vi "I_Sense_v3b.vi"(8 "error in":errorcluster, 9 "Test Freq":enum16{"10Hz", "1kHz", "20kHz"}(ring), 10 "Write Channel(s)":string="NI9264/ao2") -> (0 "error out":errorcluster, 3 "Result":dbl[](array[numeric]))   [LabVIEW 2021]
uses:
  <vilib>/DAQmx/write.llb/DAQmx Write (Analog 1D Wfm NChan NSamp).vi
  <vilib>/DAQmx/read.llb/DAQmx Read (Analog 1D Wfm NChan NSamp).vi
  <vilib>/DAQmx/create/channels.llb/DAQmx Create Channel (AO-Voltage-Basic).vi
  <vilib>/DAQmx/create/channels.llb/DAQmx Create Channel (AI-Voltage-Basic).vi
  <vilib>/DAQmx/configure/timing.llb/DAQmx Timing (Sample Clock).vi
  <vilib>/measure/mascope.llb/Amplitude and Levels N chan.vi
  <vilib>/DAQmx/miscellaneous.llb/DAQmx Fill In Error Info.vi
  <vilib>/measure/madcrms.llb/Basic Averaged DC-RMS for N Chan.vi
  <resource>/objmgr/daqmx.rc
  <vilib>/measure/NI_MABase.lvlib
  <vilib>/measure/NI_MAPro.lvlib
panel:
  in  "Cycles":i32=4
  in  "Read Channel(s)":string="BONTS_ISENSE"
  out "DC values":dbl[](array[numeric]) format="%.2p"
  out "Gains":dbl[](array[numeric])
  out "Amplitude Out":dbl[](array[numeric]) format="%.2p"
  out "High Out":dbl[](array[numeric]) format="%.2p"
  out "Low Out":dbl[](array[numeric]) format="%.2p"
  out "Amplitude In":dbl[](array[numeric]) format="%.2p"
  out "Low In":dbl[](array[numeric]) format="%.2p"
  out "High In":dbl[](array[numeric]) format="%.2p"
  in  "Sample Mode":i32(ring)=10123 items=["Finite Samples"=10178, "Continuous Samples"=10123, "Hardware Timed Single Point"=12522]
  out "Output Waveform":waveform(dbl)[](graph)=[{"t0"=timestamp(0 s since 1904-01-01), "dt"=0.001, "Y"=[]}]
  out "Input Waveform":waveform(dbl)[](graph)=[{"t0"=timestamp(0 s since 1904-01-01), "dt"=0.001, "Y"=[]}]
  in  "Sample Clock Source":tag="OnboardClock"
  out "Actual Sample Rate":dbl=1000.0 format="%0.2f"
  # "ISENSE_C+"
  # "ISENSE_C-"
  # "ISENSE_C+"
  # "ISENSE_C-"
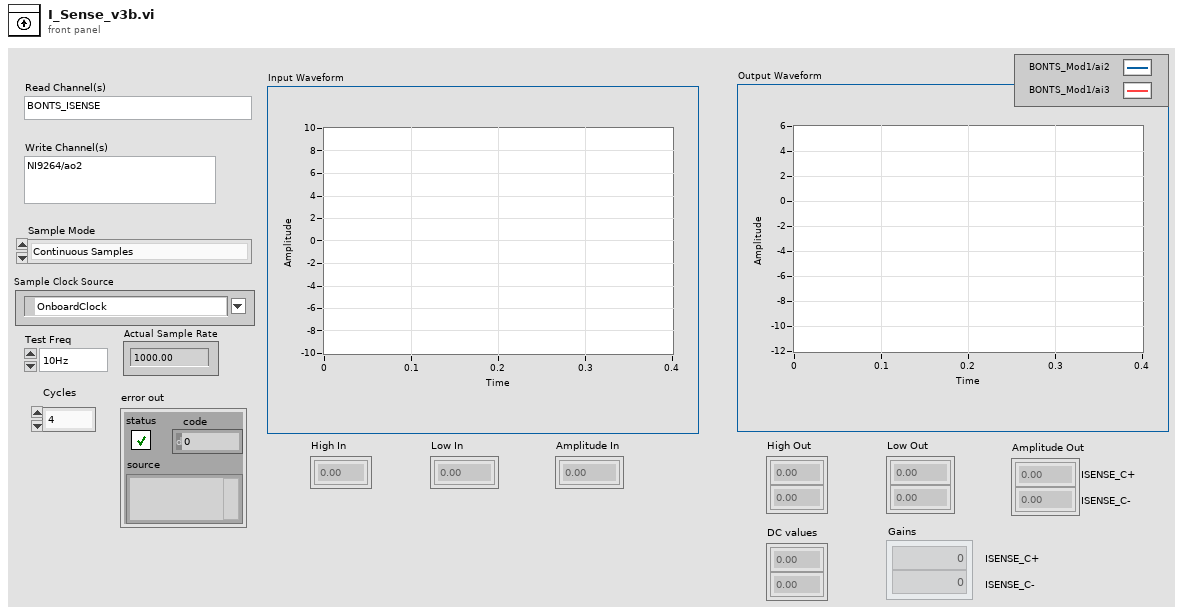
[diagram p1: front panel]
types:
  T1 = cluster{"Waveform Type":u16, "Amplitude":dbl, "Frequency":dbl}[]
  T2 = cluster{"Waveform Type":u16, "Amplitude":dbl, "Frequency":dbl}
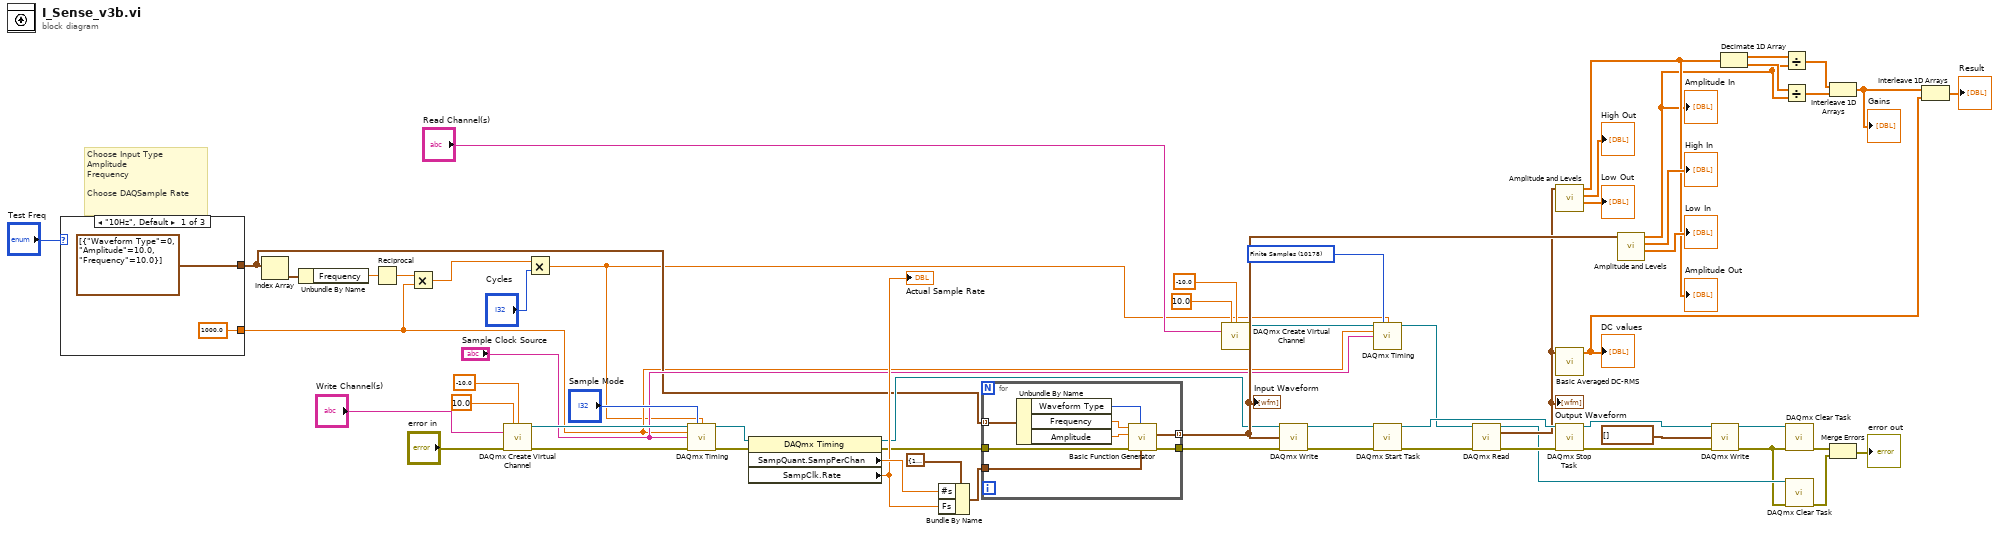
[diagram p0: block diagram]
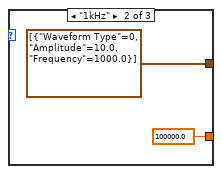
[diagram p2: hidden frame]
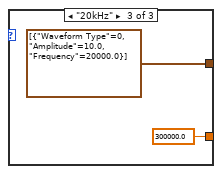
[diagram p3: hidden frame]
diagram:
  w16 = 10178 items=["Finite Samples"=10178, "Continuous Samples"=10123, "Hardware Timed Single Point"=12522] ("sample mode")
  # "Choose Input Type\nAmplitude \nFrequency\n\nChoose DAQSample Rate"
  n1 = case shown="\"10Hz\", Default" "Test Freq" {
    tunnel: [1000.0 ("Sample Rate") 100000.0 ("Sample Rate") 300000.0 ("Sample Rate")] -> w4
    tunnel: [T1 [{"Waveform Type"=0, "Amplitude"=10.0, "Frequency"=10.0}] ("Output Array") T1 [{"Waveform Type"=0, "Amplitude"=10.0, "Frequency"=1000.0}] ("Output Array") T1 [{"Waveform Type"=0, "Amplitude"=10.0, "Frequency"=20000.0}] ("Output Array")] -> w8
    frame "10Hz", Default {
    }
    frame "1kHz" {
    }
    frame "20kHz" {
    }
  }
  n2 = Index Array(array=w8) -> (element=w7:T2)  [unwired: 1 in]
  n3 = Unbundle By Name(w7) -> ("Frequency"=w6:dbl)
  n4 = Reciprocal(x=w6) -> (1/x=w5:dbl)
  n5 = Multiply(x=w5, y=w4) -> (x*y=w3:dbl)
  n6 = call-poly <vilib>:"DAQmx Create Virtual Channel.vi"("maximum value"=10.0, "minimum value"=-10.0, "physical channels"="Write Channel(s)", "error in"="error in") -> ("task out"=w58:refnum<k21>, "error out"=w59:errorcluster)  [unwired: 10 in]
  n7 = Multiply(x=w3, y="Cycles") -> (x*y=w2:dbl)
  n8 = call-poly <vilib>:"DAQmx Timing.vi"("task/channels in"=w58, "sample mode"="Sample Mode", "samples per channel"=w2, "rate"=w4, "source"="Sample Clock Source", "error in"=w59) -> ("task out"=w28:refnum<k21>, "error out"=w61:errorcluster)  [unwired: 8 in]
  n9 = property class="DAQmx Timing"(reference=w28, error in=w61) -> (reference out=w25:refnum<k21>, error out=w49:errorcluster, "SampQuant.SampPerChan"=w52:dbl, "SampClk.Rate"=w51:dbl)
  "Actual Sample Rate" <- w51
  n10 = Bundle By Name(cluster=cluster{"Fs":dbl, "#s":dbl} {"Fs"=1000.0, "#s"=1000.0} ("sampling info"), "#s"=w52, "Fs"=w51) -> (w56:cluster{"Fs":dbl, "#s":dbl})
  n11 = for {
    tunnel: w49 -> [w75]
    tunnel: w56 -> [w74]
    tunnel: [w73] -> w53
    tunnel: w8 -> [w72] mode=indexing
    tunnel: [w68] -> w44 mode=indexing
    n12 = Unbundle By Name(w72) -> ("Waveform Type"=w71:u16, "Frequency"=w70:dbl, "Amplitude"=w69:dbl)
    n13 = call <vilib>:"Basic Function Generator.vi"("sampling info"=w74, "signal type"=w71, "error in (no error)"=w75, "amplitude"=w69, "frequency"=w70) -> ("error out"=w73:errorcluster, "signal out"=w68:waveform(dbl))  [unwired: 4 in, 1 out]
  }
  "Input Waveform" <- w44
  n14 = call-poly <vilib>:"DAQmx Create Virtual Channel.vi"("maximum value"=10.0, "minimum value"=-10.0, "physical channels"="Read Channel(s)") -> ("task out"=w20:refnum<k21>)  [unwired: 11 in, 1 out]
  n15 = call-poly <vilib>:"DAQmx Write.vi"("task/channels in"=w25, "data"=w44, "error in"=w53) -> ("task out"=w55:refnum<k21>, "error out"=w54:errorcluster)  [unwired: 10 in, 1 out]
  n16 = call-poly <vilib>:"DAQmx Timing.vi"("task/channels in"=w20, "sample mode"=w16, "samples per channel"=w2, "rate"=w4, "source"="Sample Clock Source") -> ("task out"=w19:refnum<k21>)  [unwired: 9 in, 1 out]
  n17 = call <vilib>:"DAQmx Start Task.vi"("task/channels in"=w55, "error in"=w54) -> ("task out"=w50:refnum<k21>, "error out"=w48:errorcluster)  [unwired: 12 in]
  n18 = call-poly <vilib>:"DAQmx Read.vi"("task/channels in"=w19, "error in"=w48) -> ("task out"=w18:refnum<k21>, "data"=w32:waveform(dbl)[], "error out"=w47:errorcluster)  [unwired: 11 in]
  "Output Waveform" <- w32
  n19 = call-poly <vilib>:"Amplitude and Levels.vi"("signal(s) in"=w32) -> ("low state level"=→"Low Out":dbl[], "high state level"=→"High Out":dbl[], "amplitude"=w38:dbl[])  [unwired: 7 in, 1 out]
  "Amplitude Out" <- w38
  n20 = call-poly <vilib>:"Basic Averaged DC-RMS.vi"("signals in"=w32) -> ("DC values"=w30:dbl[])  [unwired: 7 in, 3 out]
  "DC values" <- w30
  n21 = call <vilib>:"DAQmx Stop Task.vi"("task/channels in"=w50, "error in"=w47) -> ("task out"=w23:refnum<k21>, "error out"=w24:errorcluster)  [unwired: 12 in]
  n22 = call-poly <vilib>:"Amplitude and Levels.vi"("signal(s) in"=w44) -> ("low state level"=→"Low In":dbl[], "high state level"=→"High In":dbl[], "amplitude"=w35:dbl[])  [unwired: 7 in, 1 out]
  "Amplitude In" <- w35
  n23 = call-poly <vilib>:"DAQmx Write.vi"("task/channels in"=w23, "data"=waveform(dbl)[] [], "error in"=w24) -> ("task out"=w22:refnum<k21>, "error out"=w17:errorcluster)  [unwired: 10 in, 1 out]
  n24 = Decimate 1D Array(w38) -> (w37:dbl[], w36:dbl[])
  n25 = Divide(x=w37, y=w35) -> (x/y=w34:dbl[])
  n26 = Divide(x=w36, y=w35) -> (x/y=w33:dbl[])
  n27 = call <vilib>:"DAQmx Clear Task.vi"("task in"=w22, "error in"=w17) -> ("error out"=w14:errorcluster)  [unwired: 13 in]
  n28 = call <vilib>:"DAQmx Clear Task.vi"("task in"=w18, "error in"=w17) -> ("error out"=w13:errorcluster)  [unwired: 13 in]
  n29 = Interleave 1D Arrays(w34, w33) -> (w31:dbl[])
  "Gains" <- w31
  n30 = Merge Errors(w14, w13) -> (→"error out":errorcluster)
  n31 = Interleave 1D Arrays(w31, w30) -> (→"Result":dbl[])
